vi "GetCurlSpeed.vi"(11 "SecondaryJoystickValues":dbl[](array[numeric])) -> (3 "Curl Speed":dbl)   [LabVIEW 2018]
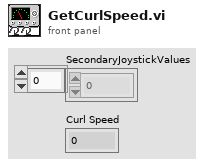
[diagram p1: front panel]
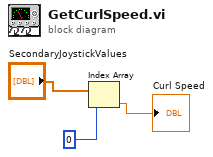
[diagram p0: block diagram]
diagram:
  n1 = Index Array(array="SecondaryJoystickValues", index=0) -> (element=→"Curl Speed":dbl)
